vi "SlowLogger_LogGEMBANK.vi"(8 "error in (no error)":errorcluster, 9 "GEM_DATA Cluster":T1, 11 "SlowLogger in":refnum<class "SlowLogger.lvclass">) -> (0 "error out":errorcluster, 1 "Dt satisfied (data logged)":bool=TRUE, 2 "Dt (s)":dbl, 3 "SlowLogger out":refnum<class "SlowLogger.lvclass">, 4 "timed out?":bool)   [LabVIEW 2018, in "feGEM DataPacker.lvlib" / "SlowLogger.lvclass"]
uses:
  SlowLogger.lvclass
  DataPacker/DataStructures/GEM_DATA_cluster_typedef.ctl
  SlowLogger.lvclass/SlowLogger.ctl
  DataPacker/ErrorTypes.ctl
  feGEM DataPacker.lvlib
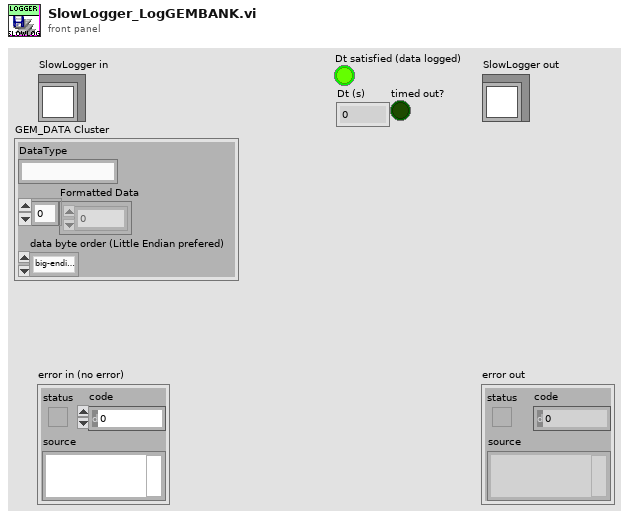
[diagram p1: front panel]
types:
  T1 = typedef "feGEM DataPacker.lvlib/GEM_DATA_cluster_typedef.ctl" = cluster{"DataType":string, "Formatted Data":u8[], "data byte order (Little Endian prefered)":enum16{"big-endian, network order", "native, host order", "little-endian"}}
  T2 = typedef "feGEM DataPacker.lvlib/GEM_BANK_CLUSTER_typedef.ctl" = cluster{"Category":string, "Variable Name":string, "Equipment description":string, "History Settings":u16, "Period to update history plots":u16, "GEM_DATA Cluster":T1}
  T3 = typedef "feGEM DataPacker.lvlib/ErrorTypes.ctl" = i32
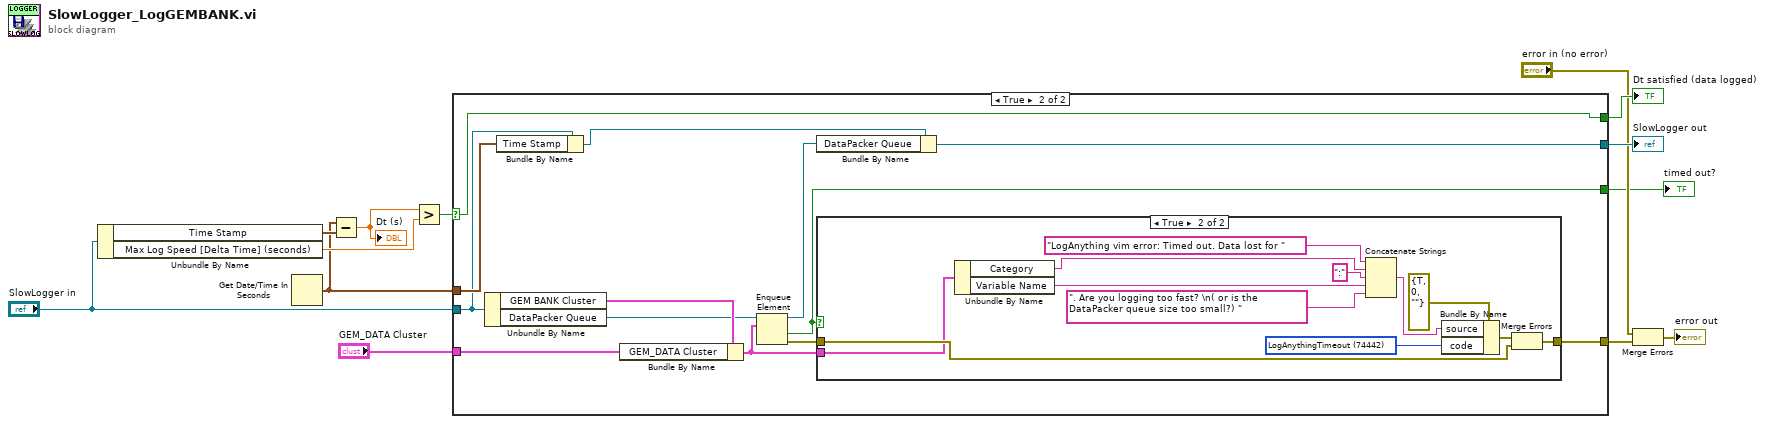
[diagram p0: block diagram]
diagram:
  n1 = Unbundle By Name("SlowLogger in") -> ("Time Stamp"=w7:timestamp, "Max Log Speed [Delta Time] (seconds)"=w9:dbl)
  n2 = Get Date/Time In Seconds() -> (seconds since 1Jan1904=w6:timestamp)
  n3 = Subtract(x=w6, y=w7) -> (x-y=w10:dbl)
  "Dt (s)" <- w10
  n4 = Greater?(x=w10, y=w9) -> (0:w8:bool)
  n5 = case shown="True" w8 {
    selector: w8 -> [w15 w28]
    tunnel: "SlowLogger in" -> [w14 w26]
    tunnel: [w15 w28] -> w11
    tunnel: w6 -> [_ w27]
    tunnel: [w14 w21] -> w12
    tunnel: [_ w23] -> w5
    tunnel: "GEM_DATA Cluster" -> [_ w17]
    tunnel: [_ w16] -> w1
    frame False {
    }
    frame True {
      n6 = Unbundle By Name(w26) -> ("GEM BANK Cluster"=w25:T2, "DataPacker Queue"=w19:refnum<queue>)
      n7 = Bundle By Name(cluster=w26, "Time Stamp"=w27) -> (w22:refnum<class "SlowLogger.lvclass">)
      n8 = Bundle By Name(cluster=w25, "GEM_DATA Cluster"=w17) -> (w18:T2)
      n9 = Enqueue Element(queue=w19, element=w18) -> (queue out=w20:refnum<queue>, timed out?=w16:bool, error out=w24:errorcluster)  [unwired: 2 in]
      n10 = Bundle By Name(cluster=w22, "DataPacker Queue"=w20) -> (w21:refnum<class "SlowLogger.lvclass">)
      n11 = case shown="True" w16 {
        tunnel: [w29 w33] -> w23
        tunnel: w24 -> [w29 w35]
        tunnel: w18 -> [_ w32]
        frame False {
        }
        frame True {
          w36 = T3 74442 items=["No Error"=0, "Network: mgNotSupported"=53, "Network: ncBadAddressErr"=54, "Network: ncInProgressErr"=55, "Network: ncTimeOutErr"=56, "Network: ncBusyErr"=57, "Network: ncNotSupportedErr"=58, "Network: ncNetErr"=59, "Network: ncAddrInUseErr"=60, "Network: ncSysOutOfMemErr"=61, "Network: ncSysOutOfMemErr"=62, "Network: ncConnRefusedErr"=63, "Network: ncAlreadyConnectedErr"=65, "Network: ncConnClosedErr"=66, "LogAnythingTimeout"=74442, "MIDAS buffer overflow!"=74443, "LVBANK CORRUPTION"=74444, "Bad Bank Name"=74445] ("Ring")
          n12 = Unbundle By Name(w32) -> ("Category"=w31:string, "Variable Name"=w30:string)
          n13 = Concatenate Strings("LogAnything vim error: Timed out. Data lost for " ("string"), w31, ":" ("string"), w30, ". Are you logging too fast? \n( or is the DataPacker queue size too small?) " ("string")) -> (w37:string)
          n14 = Bundle By Name(cluster=errorcluster {"status"=TRUE, "code"=0, "source"=""} ("error out 2"), "source"=w37, "code"=w36) -> (w34:errorcluster)
          n15 = Merge Errors(w34, w35) -> (w33:errorcluster)
        }
      }
    }
  }
  "SlowLogger out" <- w12
  "Dt satisfied (data logged)" <- w11
  "timed out?" <- w1
  n16 = Merge Errors("error in (no error)", w5) -> (→"error out":errorcluster)
